vi "CSV path to talon srx path.vi"() -> ()   [LabVIEW 2019]
uses:
  <vilib>/Rock Robotics/WPI/ThirdParty/Phoenix-LabVIEW/Motor Controller/Controls/CTRE_Phoenix_MotorControl_MotionProfileTrajectoryPoint.ctl
  <vilib>/Utility/file.llb/Read Delimited Spreadsheet (DBL).vi
panel:
  out "all rows":dbl[][](array[numeric])
  out "Motion Profile Trajectory Point Array":T1[](array[typedef])
  in  "Wheel Diameter (M)":dbl
  in  "Encoder Units":dbl
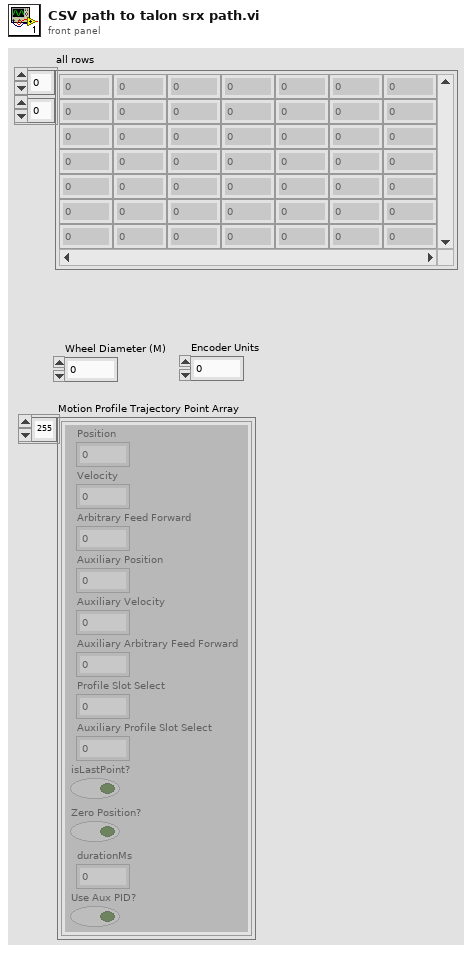
[diagram p1: front panel]
types:
  T1 = typedef "CTRE_Phoenix_MotorControl_MotionProfileTrajectoryPoint.ctl" = cluster{"Position":dbl, "Velocity":dbl, "Arbitrary Feed Forward":dbl, "Auxiliary Position":dbl, "Auxiliary Velocity":dbl, "Auxiliary Arbitrary Feed Forward":dbl, "Profile Slot Select":i32, "Auxiliary Profile Slot Select":i32, "isLastPoint?":bool, "Zero Position?":bool, "durationMs":u32, "Use Aux PID?":bool}
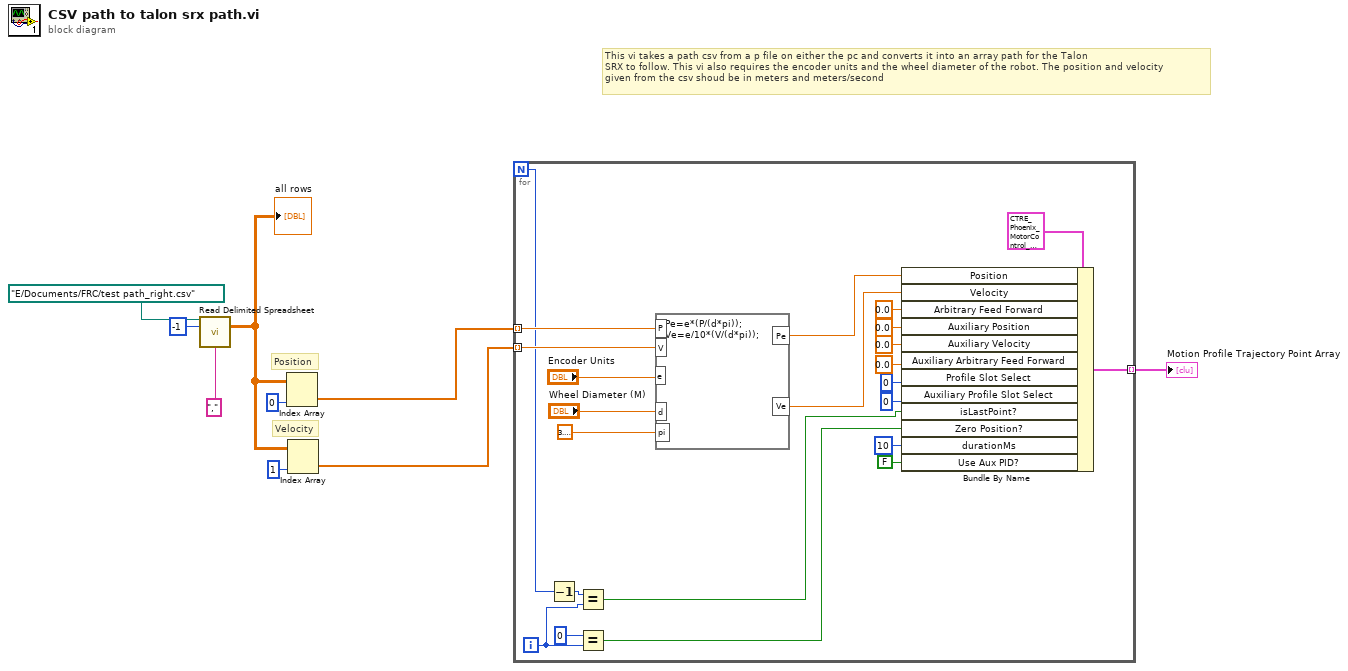
[diagram p0: block diagram]
diagram:
  # "This vi takes a path csv from a p file on either the pc and converts it into an array path for the Talon\nSRX to follow. This vi also requires the encoder units and the wheel diameter of the robot. The position and velocity\ngiven from the csv shoud be in meters and meters/second"
  # "Velocity"
  # "Position"
  n1 = call-poly <vilib>:"Read Delimited Spreadsheet.vi"("file path (dialog if empty)"=path "E:/Documents/FRC/test path_right.csv", "number of rows (all:-1)"=-1, "delimiter (\\t)"="," ("delimiter (\\t)")) -> ("all rows"=w6:dbl[][])  [unwired: 7 in, 5 out]
  "all rows" <- w6
  n2 = Index Array(array=w6, index (col)=0 ("disabled index (col)")) -> (element=w5:dbl[])  [unwired: 1 in]
  n3 = Index Array(array=w6, index (col)=1 ("index (row)")) -> (element=w4:dbl[])  [unwired: 1 in]
  n4 = for {
    N -> [w12]
    tunnel: w5 -> [w20] mode=indexing
    tunnel: w4 -> [w19] mode=indexing
    tunnel: [w17] -> w3 mode=indexing
    i -> [w11]
    n5 = Decrement(x=w12) -> (x-1=w13:i32)
    n6 = Equal?(x=w13, y=w11) -> (x = y?=w10:bool)
    n7 = Equal?(x=0, y=w11) -> (x = y?=w15:bool)
    n8 = formula code="Pe=e*(P/(d*pi));\nVe=e/10*(V/(d*pi));"("P"=w20, "d"="Wheel Diameter (M)", "pi"=3.141592653589793, "V"=w19, "e"="Encoder Units") -> ("Pe"=w29:dbl, "Ve"=w28:dbl)
    n9 = Bundle By Name(cluster=T1 {"Position"=0.0, "Velocity"=0.0, "Arbitrary Feed Forward"=0.0, "Auxiliary Position"=0.0, "Auxiliary Velocity"=0.0, "Auxiliary Arbitrary Feed Forward"=0.0, "Profile Slot Select"=0, "Auxiliary Profile Slot Select"=0, "isLastPoint?"=FALSE, "Zero Position?"=FALSE, "durationMs"=0, "Use Aux PID?"=FALSE} ("Trajectory Point"), "Position"=w29, "Velocity"=w28, "Arbitrary Feed Forward"=0.0, "Auxiliary Position"=0.0, "Auxiliary Velocity"=0.0, "Auxiliary Arbitrary Feed Forward"=0.0, "Profile Slot Select"=0, "Auxiliary Profile Slot Select"=0, "isLastPoint?"=w10, "Zero Position?"=w15, "durationMs"=u32 10, "Use Aux PID?"=FALSE) -> (w17:T1)
  }
  "Motion Profile Trajectory Point Array" <- w3
